vi "DrawBGtiles.vi"(4 "y":u16, 6 "x":u16, 7 "Tilebuffer":refnum<k21>="TileBuffer", 11 "color_in":fxp<+,3,3>) -> (3 "color_out":fxp<+,3,3>)   [LabVIEW 2019, in "GameEngine.lvlib"]
uses:
  GameEngine.lvlib
  <vilib>/rvi/Memory/Memory_Emulation/nirvimemoryFastEmulation.vi
  <vilib>/rvi/Memory/Memory_Emulation/nirvimemoryEmulation.vi
  <vilib>/rvi/Emulation/niFpgaEmulationIsFPGAContextNoSignature.vi
  <vilib>/rvi/DataTransferAndStorage/Container/Common/niFpgaContainerGetUniqueNameForEmu.vi
  <vilib>/rvi/Emulation/niFpgaProcessEmulError.vi
  <vilib>/rvi/Emulation/niFpgaSctlEmulationGetInTimedLoop.vi
  <vilib>/rvi/errors/nirviReportUnexpectedCaseInternalError (U32).vi
  <vilib>/rvi/DataTransferAndStorage/Container/XNode/niFpgaContainer.xnode
  Tiles/Tiles.lvlib
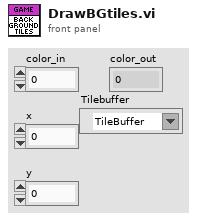
[diagram p1: front panel]
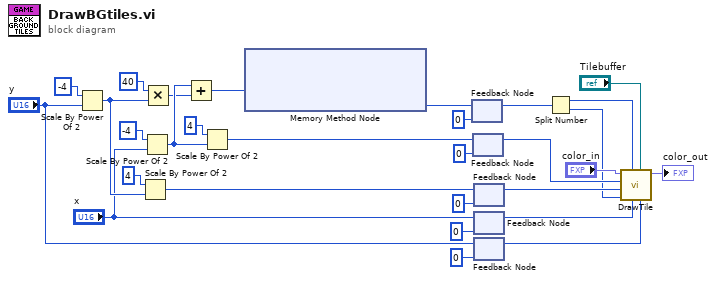
[diagram p0: block diagram]
diagram:
  n1 = Scale By Power Of 2(n=i16 -4, x="y") -> (x*2^n=w24:u16)
  n2 = Scale By Power Of 2(n=i16 4, x=w24) -> (x*2^n=w25:u16)
  n3 = Scale By Power Of 2(n=i16 -4, x="x") -> (x*2^n=w21:u16)
  n4 = Multiply(x=u16 40, y=w24) -> (x*y=w8:u16)
  n5 = Add(x=w21, y=w8) -> (x+y=w18:u16)
  n6 = Scale By Power Of 2(n=i16 4, x=w21) -> (x*2^n=w22:u16)
  n7 = xnode ("Memory Method Node")("Address"=w18) -> ("Data"=w19:u16)  [unwired: 1 in, 1 out]
  n8 = feedback #1(u16 0 ("Data")) -> (w27:u16)
  n9 = feedback-in #1(w19) -> ()
  n10 = feedback #2(u16 0) -> (w12:u16)
  n11 = feedback-in #2(w22) -> ()
  n12 = feedback #3(u16 0) -> (w11:u16)
  n13 = feedback-in #3(w25) -> ()
  n14 = feedback #4(u16 0 ("x")) -> (w10:u16)
  n15 = feedback-in #4("x") -> ()
  n16 = feedback #5(u16 0 ("y")) -> (w9:u16)
  n17 = feedback-in #5("y") -> ()
  n18 = Split Number(x=w27) -> (hi(x)=w2:u8, lo(x)=w1:u8)
  n19 = call "DrawTile.vi"("index_y"=w9, "Tilebuffer"="Tilebuffer", "index_x"=w10, "TileNo"=w2, "Rotate"=w1, "pos_y"=w11, "pos_x"=w12, "color_in"="color_in") -> ("color_out"=→"color_out":fxp<+,3,3>)  [unwired: 3 in]
